vi "AVTCP-Server.vi"() -> ()   [LabVIEW 2020]
uses:
  Sub VIs/AVTCP-FGV Action.ctl
  epl-vi-lib/epl-network/Source/epl-network.lvlib
panel:
  in  "Cancel":bool
  out "finished":errorcluster
  in  "start":bool
  out "Port":i32
  out "IP Address":string
  in  "stop":bool
  out "Ready":bool caption="Wait: Initializing hardware..."
  out "Client":bool
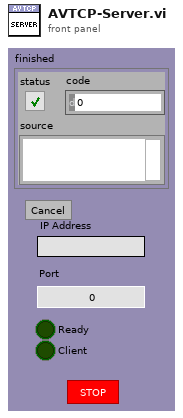
[diagram p1: front panel]
types:
  T1 = typedef "epl-network.lvlib/IPEndPoint.ctl" = cluster{"address":string, "port":i32}
  T2 = enum8{"Enabled", "Disabled", "Disabled and Grayed Out"}
  T3 = typedef "AVTCP-FGV Action.ctl" = enum16{"Init", "Write", "Read"}
  T4 = typedef "epl-network.lvlib/TCP Message.ctl" = cluster{"Code":i32, "Command":string, "Payload":string}
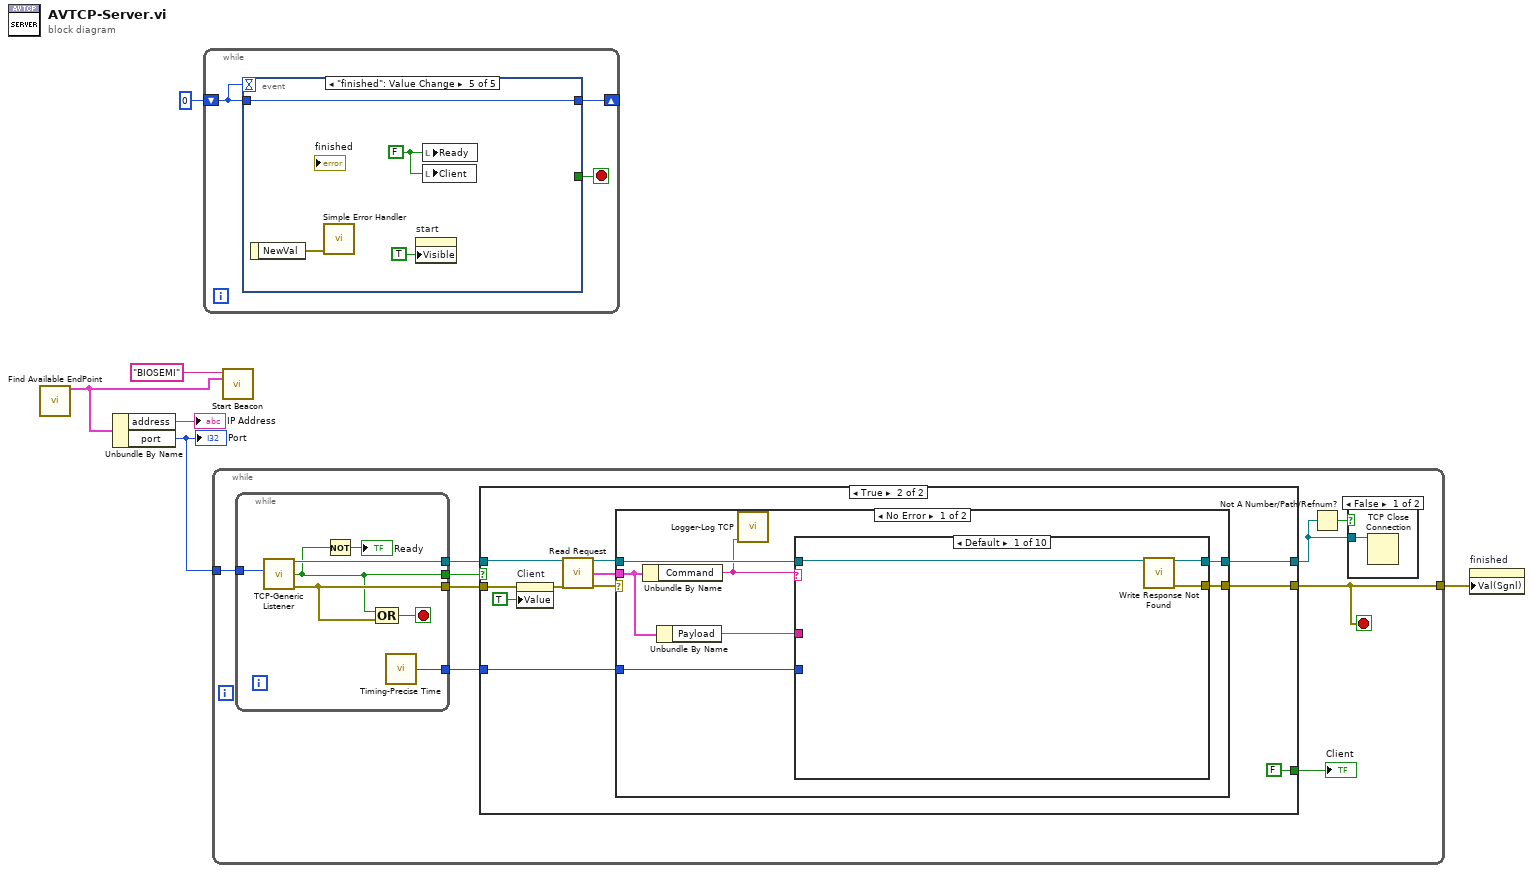
[diagram p0: block diagram]
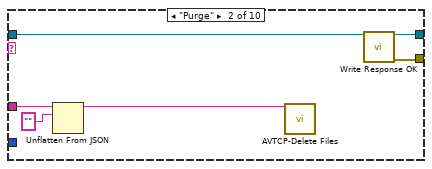
[diagram p3: hidden frame]
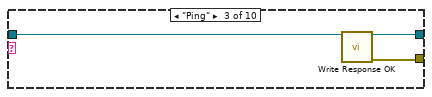
[diagram p4: hidden frame]
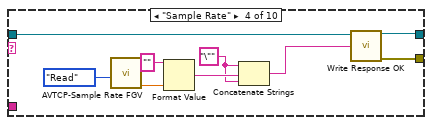
[diagram p5: hidden frame]
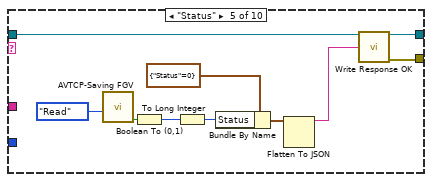
[diagram p6: hidden frame]
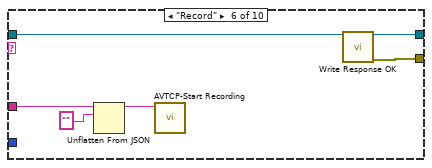
[diagram p7: hidden frame]
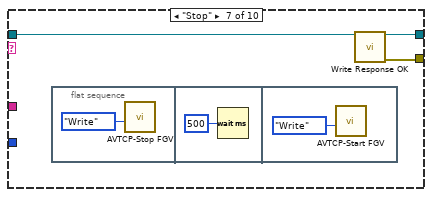
[diagram p8: hidden frame]
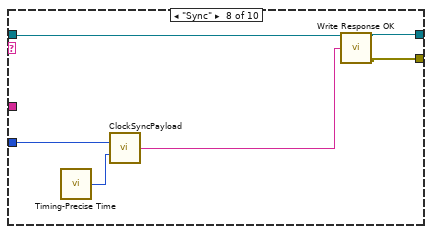
[diagram p9: hidden frame]
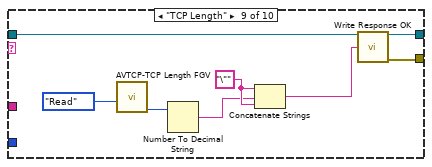
[diagram p10: hidden frame]
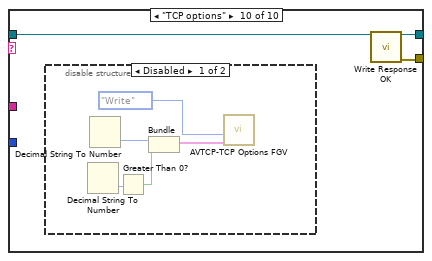
[diagram p11: hidden frame]
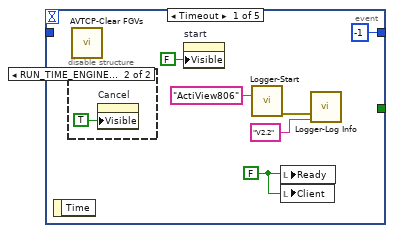
[diagram p15: hidden frame]
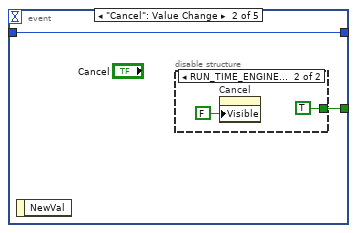
[diagram p17: hidden frame]
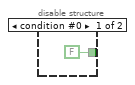
[diagram p18: hidden frame]
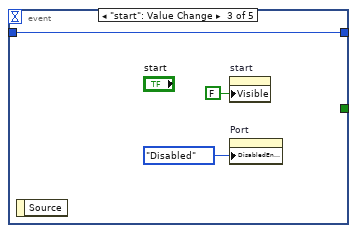
[diagram p19: hidden frame]
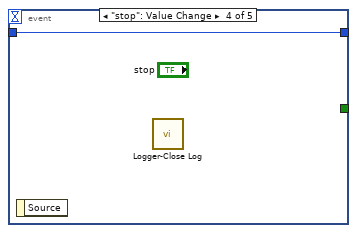
[diagram p20: hidden frame]
diagram:
  n1 = call "Find Available EndPoint.vi"() -> ("IPEndPoint"=w3:T1)  [unwired: 14 in, 1 out]
  n2 = Unbundle By Name(w3) -> ("address"=→"IP Address":string, "port"=w1:i32)
  "Port" <- w1
  n3 = while {
    shift-right: [w8] -> _
    shift-left: 0 -> [w7]
    stop <- w9 stop-if-true
    n4 = event shown="[4] \"finished\": Value Change" {
      selector: _ -> [_ _ _ _ _]
      dyn-events: _ -> [_ _ _ _ _]
      timeout: w7 -> [_ _ _ _ _]
      tunnel: [_ w17 _ _ _] -> w9
      tunnel: [-1 w18 w24 w25 w29] -> w8
      tunnel: w7 -> [_ w18 w24 w25 w29]
      event Timeout {
        w14 = FALSE
        n5 = event-data() -> ()  [unwired: 1 in, 1 out]
        n6 = disable-structure shown="RUN_TIME_ENGINE==False" {
          frame condition #0 {
          }
          frame condition #1 (active) {
            n7 = property on="Cancel" class="Bool"("Visible"=TRUE) -> ()  [unwired: 2 in, 2 out]
          }
        }
        n8 = call "AVTCP-Clear FGVs.vi"() -> ()  [unwired: 12 in]
        n9 = property on="start" class="Bool"("Visible"=FALSE) -> ()  [unwired: 2 in, 2 out]
        n10 = call "Logger-Start.vi"("Name"="ActiView806") -> ("error out"=w11:errorcluster)  [unwired: 14 in]
        n11 = local write "Ready"(w14) -> ()
        n12 = local write "Client"(w14) -> ()
        n13 = call "Logger-Log Info.vi"("error in (no error)"=w11, "Message"="V2.2") -> ()  [unwired: 13 in, 1 out]
      }
      event "Cancel": Value Change {
        n14 = event-data() -> ()  [unwired: 1 in, 1 out]
        n15 = disable-structure shown="RUN_TIME_ENGINE==False" {
          disable-tunnel: [FALSE TRUE] -> w17
          frame condition #0 {
          }
          frame condition #1 (active) {
            n16 = property on="Cancel" class="Bool"("Visible"=FALSE) -> ()  [unwired: 2 in, 2 out]
          }
        }
      }
      event "start": Value Change {
        n17 = event-data() -> ()  [unwired: 1 in, 1 out]
        n18 = property on="start" class="Bool"("Visible"=FALSE) -> ()  [unwired: 2 in, 2 out]
        n19 = property on="Port" class="DigNum (strict)"("DisabledEnum"=T2."Disabled" ("Disabled")) -> ()  [unwired: 2 in, 2 out]
      }
      event "stop": Value Change {
        n20 = event-data() -> ()  [unwired: 1 in, 1 out]
        n21 = call "Logger-Close Log.vi"() -> ()  [unwired: 15 in, 1 out]
      }
      event "finished": Value Change {
        w28 = FALSE ("Ready")
        n22 = event-data() -> ("NewVal"=w27:errorcluster)  [unwired: 1 in]
        n23 = call <vilib>:"Simple Error Handler.vi"("error in (no error)"=w27) -> ()  [unwired: 4 in, 5 out]
        n24 = property on="start" class="Bool"("Visible"=TRUE) -> ()  [unwired: 2 in, 2 out]
        n25 = local write "Ready"(w28) -> ()
        n26 = local write "Client"(w28) -> ()
      }
    }
  }
  n27 = while {
    tunnel: w1 -> [w34]
    tunnel: [w31] -> w5
    stop <- w31 stop-if-true
    n28 = while {
      tunnel: [w41] -> w38
      tunnel: [w45] -> w37
      tunnel: w34 -> [w40]
      tunnel: [w43] -> w33
      tunnel: [w39] -> w30
      stop <- w44 stop-if-true
      n29 = call "TCP-Generic Listener.vi"("port"=w40) -> ("connection ID"=w45:refnum<k5>, "Connected?"=w41:bool, "error out"=w43:errorcluster)  [unwired: 12 in]
      n30 = Not(x=w41) -> (.not. x?=→"Ready":bool)
      n31 = Compound Arithmetic op=OR(w41, w43) -> (w44:bool)
      n32 = call "Timing-Precise Time.vi"() -> ("preciseTime"=w39:i64)  [unwired: 14 in, 1 out]
    }
    n33 = case shown="True" w38 {
      tunnel: w33 -> [w46 w57]
      tunnel: w37 -> [w47 w52]
      tunnel: [w47 w55] -> w35
      tunnel: [w46 w54] -> w31
      tunnel: [_ FALSE] -> w32
      tunnel: w30 -> [_ w53]
      frame False {
      }
      frame True {
        n34 = property on="Client" class="Bool (strict)"(error in=w57, "Value"=TRUE ("Client")) -> (error out=w51:errorcluster)  [unwired: 1 in, 1 out]
        n35 = call "Read Request.vi"("connection ID"=w52, "error in (no error)"=w51) -> ("connection ID out"=w49:refnum<k5>, "TCPMessage"=w48:T4, "error out"=w50:errorcluster)  [unwired: 11 in]
        n36 = case shown="No Error" w50 {
          selector: w50 -> [_ w131]
          tunnel: w49 -> [w65 w132]
          tunnel: [w64 w132] -> w55
          tunnel: [w63 w131] -> w54
          tunnel: w53 -> [w62 _]
          tunnel: w48 -> [w60 _]
          frame No Error {
            n37 = Unbundle By Name(w60) -> ("Command"=w61:string)
            n38 = Unbundle By Name(w60) -> ("Payload"=w59:string)
            n39 = call "Logger-Log TCP.vi"("Message"=w61) -> ()  [unwired: 14 in, 1 out]
            n40 = case shown="Default" w61 {
              tunnel: w65 -> [w66 w71 w75 w84 w91 w97 w103 w112 w115 w123]
              tunnel: [w68 w70 w77 w83 w93 w99 w105 w111 w118 w125] -> w64
              tunnel: [w67 w69 w76 w82 w92 w98 w104 w110 w117 w124] -> w63
              tunnel: w62 -> [_ _ _ _ _ _ _ w113 _ _]
              tunnel: w59 -> [_ w74 _ _ _ w101 _ _ _ _]
              frame Default {
                n41 = call "Write Response Not Found.vi"("connection ID"=w66) -> ("connection ID out"=w68:refnum<k5>, "error out"=w67:errorcluster)  [unwired: 13 in]
              }
              frame "Purge" {
                n42 = Unflatten From JSON(JSON string=w74, type and defaults="") -> (value=w72:string)  [unwired: 5 in, 1 out]
                n43 = call "AVTCP-Delete Files.vi"("Folder"=w72) -> ()  [unwired: 14 in, 1 out]
                n44 = call "Write Response OK.vi"("connection ID"=w71) -> ("connection ID out"=w70:refnum<k5>, "error out"=w69:errorcluster)  [unwired: 13 in]
              }
              frame "Ping" {
                n45 = call "Write Response OK.vi"("connection ID"=w75) -> ("connection ID out"=w77:refnum<k5>, "error out"=w76:errorcluster)  [unwired: 13 in]
              }
              frame "Sample Rate" {
                w79 = "\""
                n46 = call "AVTCP-Sample Rate FGV.vi"("Action"=AVTCP-FGV_Action."Read") -> ("Value out"=w85:dbl)  [unwired: 6 in]
                n47 = Format Value(string ("")="", value (0)=w85) -> (output string=w80:string)  [unwired: 1 in]
                n48 = Concatenate Strings(w79, w80, w79) -> (w78:string)
                n49 = call "Write Response OK.vi"("connection ID"=w84, "Payload"=w78) -> ("connection ID out"=w83:refnum<k5>, "error out"=w82:errorcluster)  [unwired: 12 in]
              }
              frame "Status" {
                n50 = call "AVTCP-Saving FGV.vi"("Action"=AVTCP-FGV_Action."Read") -> ("Value out"=w95:bool)  [unwired: 6 in]
                n51 = Boolean To (0,1)(Boolean=w95) -> (0, 1=w94:i16)
                n52 = To Long Integer(number=w94) -> (32bit integer=w89:i32)
                n53 = Bundle By Name(cluster=cluster{"Status":i32} {"Status"=0}, "Status"=w89) -> (w88:cluster{"Status":i32})
                n54 = Flatten To JSON(anything=w88) -> (JSON string=w87:string)  [unwired: 2 in, 1 out]
                n55 = call "Write Response OK.vi"("connection ID"=w91, "Payload"=w87) -> ("connection ID out"=w93:refnum<k5>, "error out"=w92:errorcluster)  [unwired: 12 in]
              }
              frame "Record" {
                n56 = Unflatten From JSON(JSON string=w101, type and defaults="") -> (value=w100:string)  [unwired: 5 in, 1 out]
                n57 = call "AVTCP-Start Recording.vi"("filepath"=w100) -> ()  [unwired: 11 in]
                n58 = call "Write Response OK.vi"("connection ID"=w97) -> ("connection ID out"=w99:refnum<k5>, "error out"=w98:errorcluster)  [unwired: 13 in]
              }
              frame "Stop" {
                n59 = flat-sequence {
                  frame #0 {
                    n60 = call "AVTCP-Stop FGV.vi"("Action"=AVTCP-FGV_Action."Write") -> ()  [unwired: 6 in, 1 out]
                  }
                  frame #1 {
                    n61 = Wait (ms)(milliseconds to wait=u32 500) -> ()  [unwired: 1 out]
                  }
                  frame #2 {
                    n62 = call "AVTCP-Start FGV.vi"("Action"=AVTCP-FGV_Action."Write") -> ()  [unwired: 6 in, 1 out]
                  }
                }
                n63 = call "Write Response OK.vi"("connection ID"=w103) -> ("connection ID out"=w105:refnum<k5>, "error out"=w104:errorcluster)  [unwired: 13 in]
              }
              frame "Sync" {
                n64 = call "Timing-Precise Time.vi"() -> ("preciseTime"=w114:i64)  [unwired: 14 in, 1 out]
                n65 = call "ClockSyncPayload.vi"("T1"=w113, "T2"=w114) -> ("JSON string"=w109:string)  [unwired: 13 in]
                n66 = call "Write Response OK.vi"("connection ID"=w112, "Payload"=w109) -> ("connection ID out"=w111:refnum<k5>, "error out"=w110:errorcluster)  [unwired: 12 in]
              }
              frame "TCP Length" {
                w121 = "\""
                n67 = call "AVTCP-TCP Length FGV.vi"("Action"=AVTCP-FGV_Action."Read") -> ("Value out"=w120:i32)  [unwired: 6 in]
                n68 = Number To Decimal String(number=w120) -> (decimal integer string=w119:string)  [unwired: 1 in]
                n69 = Concatenate Strings(w121, w119, w121) -> (w116:string)
                n70 = call "Write Response OK.vi"("connection ID"=w115, "Payload"=w116) -> ("connection ID out"=w118:refnum<k5>, "error out"=w117:errorcluster)  [unwired: 12 in]
              }
              frame "TCP options" {
                n71 = disable-structure shown="Disabled" {
                  frame Disabled {
                    n72 = Decimal String To Number() -> (number=w129:i32)  [unwired: 3 in, 1 out]
                    n73 = Decimal String To Number() -> (number=w126:i32)  [unwired: 3 in, 1 out]
                    n74 = Greater Than 0?(x=w129) -> (x > 0?=w128:bool)
                    n75 = Bundle(w126, w128) -> (w130:cluster{i32, bool})  [unwired: 1 in]
                    n76 = call "AVTCP-TCP Options FGV.vi"("Value in"=w130, "Action"=AVTCP-FGV_Action."Write") -> ()  [unwired: 4 in, 2 out]
                  }
                  frame Enabled {
                  }
                }
                n77 = call "Write Response OK.vi"("connection ID"=w123) -> ("connection ID out"=w125:refnum<k5>, "error out"=w124:errorcluster)  [unwired: 13 in]
              }
            }
          }
          frame Error {
          }
        }
      }
    }
    "Client" <- w32
    n78 = Not A Number/Path/Refnum?(number/path/refnum=w35) -> (NaN/Path/Refnum?=w36:bool)
    n79 = case shown="False" w36 {
      tunnel: w35 -> [w133 _]
      frame False {
        n80 = TCP Close Connection(connection ID=w133) -> ()  [unwired: 2 in, 2 out]
      }
      frame True {
      }
    }
  }
  n81 = call "Start Beacon.vi"("name"="BIOSEMI" ("Name"), "TCP Server EndPoint"=w3) -> ()  [unwired: 13 in, 1 out]
  n82 = property on="finished" class="Clust (strict)"("Val(Sgnl)"=w5) -> ()  [unwired: 2 in, 2 out]
